vi "Pfeiffer_DPG_202_Pressure_Readout_Continious.vi"() -> ()   [LabVIEW 2015]
uses:
  Pfeiffer Vacuum/Public/DigiLine/Digiline - Cluster.ctl
  <vilib>/Utility/file.llb/Write Delimited Spreadsheet (DBL).vi
  Pfeiffer Vacuum/Pfeiffer Vacuum.lvlib
panel:
  in  "Readout Frequency (Hz)":dbl=1.0
  out "XY Graph":cluster{"Time Array OUT":dbl[], dbl[]}[](graph)
  in  "Comments":string
  out "Scan Number":i32
  in  "stop":bool
  out "error out":errorcluster
  out "Pressure Ch 2":string
  out "Pressure Ch 1":string
  in  "Ch 2":u16=2 max=999 step=1
  in  "Ch 1":u16=1 max=999 step=1
  in  "VISA session in":refnum<visa-resource-name>="COM3"
  in  "DigiLine-Cluster":T1={"Parameter"=0, "Parameter\nread only<->describe"=FALSE, "Correction faktor\n(0,20 - 9,90) "=1.0, "Pressure set point (mbar)\n0 ==> ur (p<1,0e-4 mbar)\n1 - 2050 mbar"=0} {"Pressure set point (mbar)\n0 ==> ur (p<1,0e-4 mbar)\n1 - 2050 mbar" min=0 max=2050 step=1; "Correction faktor\n(0,20 - 9,90)" min=0.2 max=9.9 step=0.01 format="%.2f"; "Parameter" items=[" Pressure  [mbar]", " Correction factor 1", " Correction factor 2 (Bayard Albert)", " Actual error code (read only)", " Software version Transmitter  (read only)", " Unit type Transmitter (read only)"]}
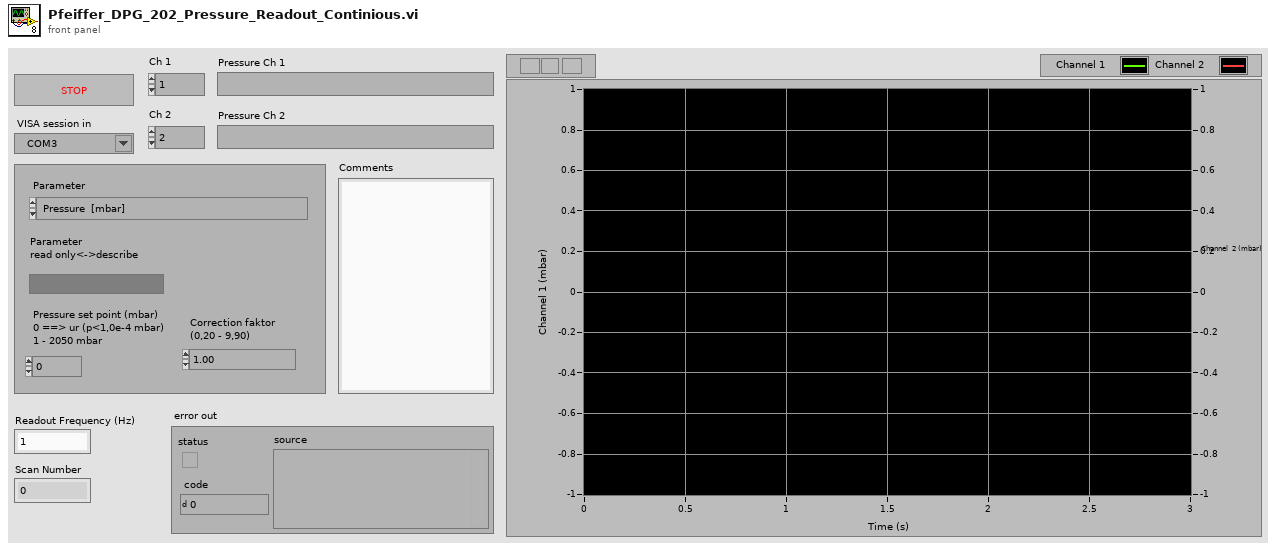
[diagram p1: front panel]
types:
  T1 = typedef "Pfeiffer Vacuum.lvlib/Digiline - Cluster.ctl" = cluster{"Parameter":u16, "Parameter\nread only<->describe":bool, "Correction faktor\n(0,20 - 9,90) ":sgl, "Pressure set point (mbar)\n0 ==> ur (p<1,0e-4 mbar)\n1 - 2050 mbar":i16}
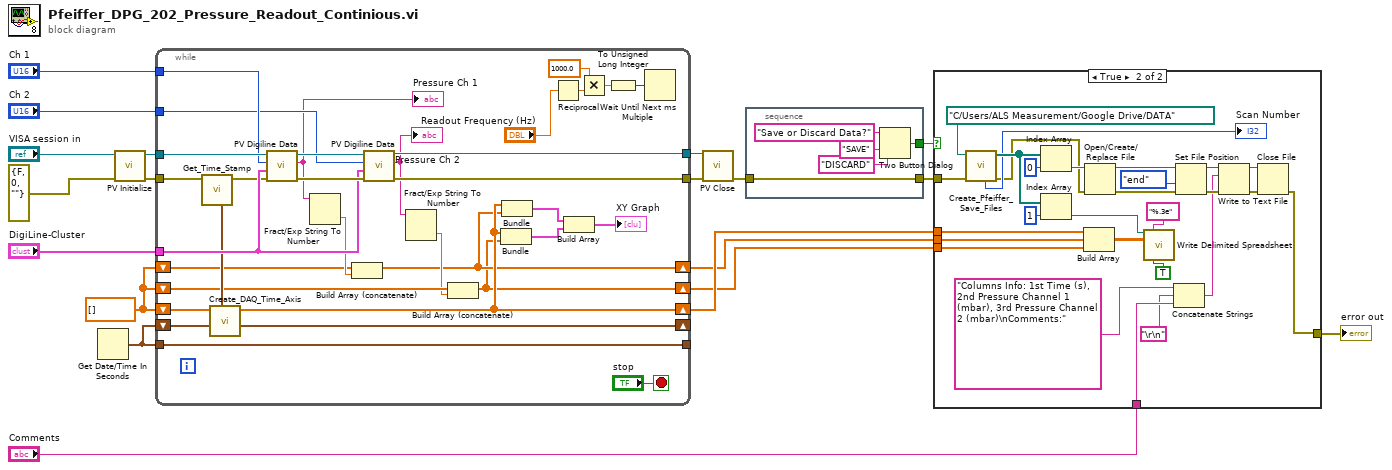
[diagram p0: block diagram]
diagram:
  w8 = dbl[] [] ("Time Array OUT")
  n1 = Get Date/Time In Seconds() -> (seconds since 1Jan1904=w9:timestamp)
  n2 = call "PV Initialize.vi"("error in (no error)"=errorcluster {"status"=FALSE, "code"=0, "source"=""}, "VISA session in"="VISA session in") -> ("error out"=w19:errorcluster, "VISA session out"=w18:refnum<visa-resource-name>)  [unwired: 8 in]
  n3 = while {
    tunnel: w19 -> [w43]
    tunnel: w18 -> [w52]
    tunnel: "Ch 1" -> [w51]
    tunnel: [w48] -> w15
    tunnel: [w47] -> w14
    tunnel: "Ch 2" -> [w46]
    tunnel: "DigiLine-Cluster" -> [w45]
    shift-right: [w30] -> w3
    shift-left: w8 -> [w40]
    shift-right: [w38] -> _
    shift-left: w9 -> [w41]
    shift-right: [w29] -> w2
    shift-left: w8 -> [w35]
    tunnel: w9 -> [w34]
    tunnel: [w34] -> _
    shift-right: [w28] -> w1
    shift-left: w8 -> [w33]
    stop <- "stop" stop-if-true
    n4 = call "Get_Time_Stamp.vi"("error in"=w43) -> ("error out"=w42:errorcluster, "current time"=w39:timestamp)  [unwired: 9 in]
    n5 = call "Create_DAQ_Time_Axis.vi"("Time Stamp Current Iteration"=w39, "Time Stamp Last Iteration"=w41, "Time Array IN"=w40) -> ("Time Stamp Current Iteration"=w38:timestamp, "Time Array OUT"=w30:dbl[])  [unwired: 6 in, 1 out]
    n6 = call "PV Digiline Data.vi"("error in (no error)"=w42, "DigiLine-Cluster"=w45, "Adress of unit"=w51, "VISA session"=w52) -> ("error out"=w49:errorcluster, "response (data)"=w37:string, "dup VISA session"=w50:refnum<visa-resource-name>)  [unwired: 5 in]
    "Pressure Ch 1" <- w37
    n7 = Fract/Exp String To Number(string=w37) -> (number=w36:dbl)  [unwired: 3 in, 1 out]
    n8 = Build Array (concatenate)(w35, w36) -> (w29:dbl[])
    n9 = call "PV Digiline Data.vi"("error in (no error)"=w49, "DigiLine-Cluster"=w45, "Adress of unit"=w46, "VISA session"=w50) -> ("error out"=w47:errorcluster, "response (data)"=w32:string, "dup VISA session"=w48:refnum<visa-resource-name>)  [unwired: 5 in]
    "Pressure Ch 2" <- w32
    n10 = Fract/Exp String To Number(string=w32) -> (number=w31:dbl)  [unwired: 3 in, 1 out]
    n11 = Build Array (concatenate)(w33, w31) -> (w28:dbl[])
    n12 = Bundle("Time Array OUT"=w30, w28) -> (w26:cluster{"Time Array OUT":dbl[], dbl[]})  [unwired: 1 in]
    n13 = Bundle("Time Array OUT"=w30, w29) -> (w27:cluster{"Time Array OUT":dbl[], dbl[]})  [unwired: 1 in]
    n14 = Reciprocal(x="Readout Frequency (Hz)") -> (1/x=w22:dbl)
    n15 = Build Array(w27, w26) -> (→"XY Graph":cluster{"Time Array OUT":dbl[], dbl[]}[])
    n16 = Multiply(x=1000.0, y=w22) -> (x*y=w21:dbl)
    n17 = To Unsigned Long Integer(number=w21) -> (unsigned 32bit integer=w24:u32)
    n18 = Wait Until Next ms Multiple(millisecond multiple=w24) -> ()  [unwired: 1 out]
  }
  n19 = call "PV Close.vi"("VISA session"=w15, "error in (no error)"=w14) -> ("error out"=w7:errorcluster)  [unwired: 13 in]
  n20 = stacked-sequence {
    tunnel: [w57] -> w11
    tunnel: w7 -> [w53]
    tunnel: [w53] -> w10
    frame #0 {
      n21 = Two Button Dialog(message="Save or Discard Data?", 1:"DISCARD" ("F button name (\"Cancel\")"), 2:"SAVE" ("T button name (\"OK\")")) -> (T button?=w57:bool)
    }
  }
  n22 = case shown="True" w11 {
    tunnel: w10 -> [w58 w62]
    tunnel: [w58 w71] -> w6
    tunnel: "Comments" -> [_ w69]
    tunnel: w3 -> [_ w66]
    tunnel: w2 -> [_ w65]
    tunnel: w1 -> [_ w64]
    frame False {
    }
    frame True {
      n23 = call "Create_Pfeiffer_Save_Files.vi"("error in (no error)"=w62, "base path"=path "C:/Users/ALS Measurement/Google Drive/DATA" ("file path (use dialog)")) -> ("error out"=w59:errorcluster, "Save Files Array"=w61:path[], "Scan Number"=→"Scan Number":i32)  [unwired: 5 in, 2 out]
      n24 = Index Array(array=w61, index=0) -> (element=w79:path)
      n25 = Index Array(array=w61, index=1) -> (element=w80:path)
      n26 = Build Array(w66, w65, w64) -> (w83:dbl[][])
      n27 = Open/Create/Replace File(file path (use dialog)=w79, error in=w59) -> (refnum out=w78:refnum<file>, error out=w75:errorcluster)  [unwired: 4 in, 1 out]
      n28 = call-poly <vilib>:"Write Delimited Spreadsheet.vi"("file path (dialog if empty)"=w80, "format (%.3f)"="%.3e", "2D data"=w83, "transpose? (F)"=TRUE ("transpose? (no:F)")) -> ()  [unwired: 10 in, 2 out]
      n29 = Concatenate Strings("Columns Info: 1st Time (s), 2nd Pressure Channel 1 (mbar), 3rd Pressure Channel 2 (mbar)\nComments:" ("text"), "\r\n", w69) -> (w70:string)
      n30 = Set File Position(refnum=w78, from (0:start)=enum16{"start", "end", "current"}."end", error in=w75) -> (refnum out=w77:refnum<file>, error out=w74:errorcluster)  [unwired: 1 in]
      n31 = Write to Text File(file (use dialog)=w77, text=w70, error in=w74) -> (refnum out=w76:refnum<file>, error out=w73:errorcluster)  [unwired: 1 in, 1 out]
      n32 = Close File(refnum=w76, error in=w73) -> (error out=w71:errorcluster)  [unwired: 1 out]
    }
  }
  "error out" <- w6
